vi "Producer Consumer Template.vi"   [LabVIEW 2020, in "Publisher Subscriber.lvlib"]
uses:
  Publisher Subscriber.lvlib
  Controls/node refnum.ctl
  Controls/data cluster.ctl
  37c060d3-9079-425a-9318-d9bb7186e347.vi
  ae88ff53-e2b6-4b5a-85aa-5b466751ef77.vi
types:
  T1 = typedef "Publisher Subscriber.lvlib/node refnum.ctl" = refnum<k1>
  T2 = cluster{"Node Ref":T1, "E Ref":refnum<event-registration>, "Message":string, "Tout":i32}
  T3 = cluster{"Node Ref":T1, "Message":string, "Tout":i32}
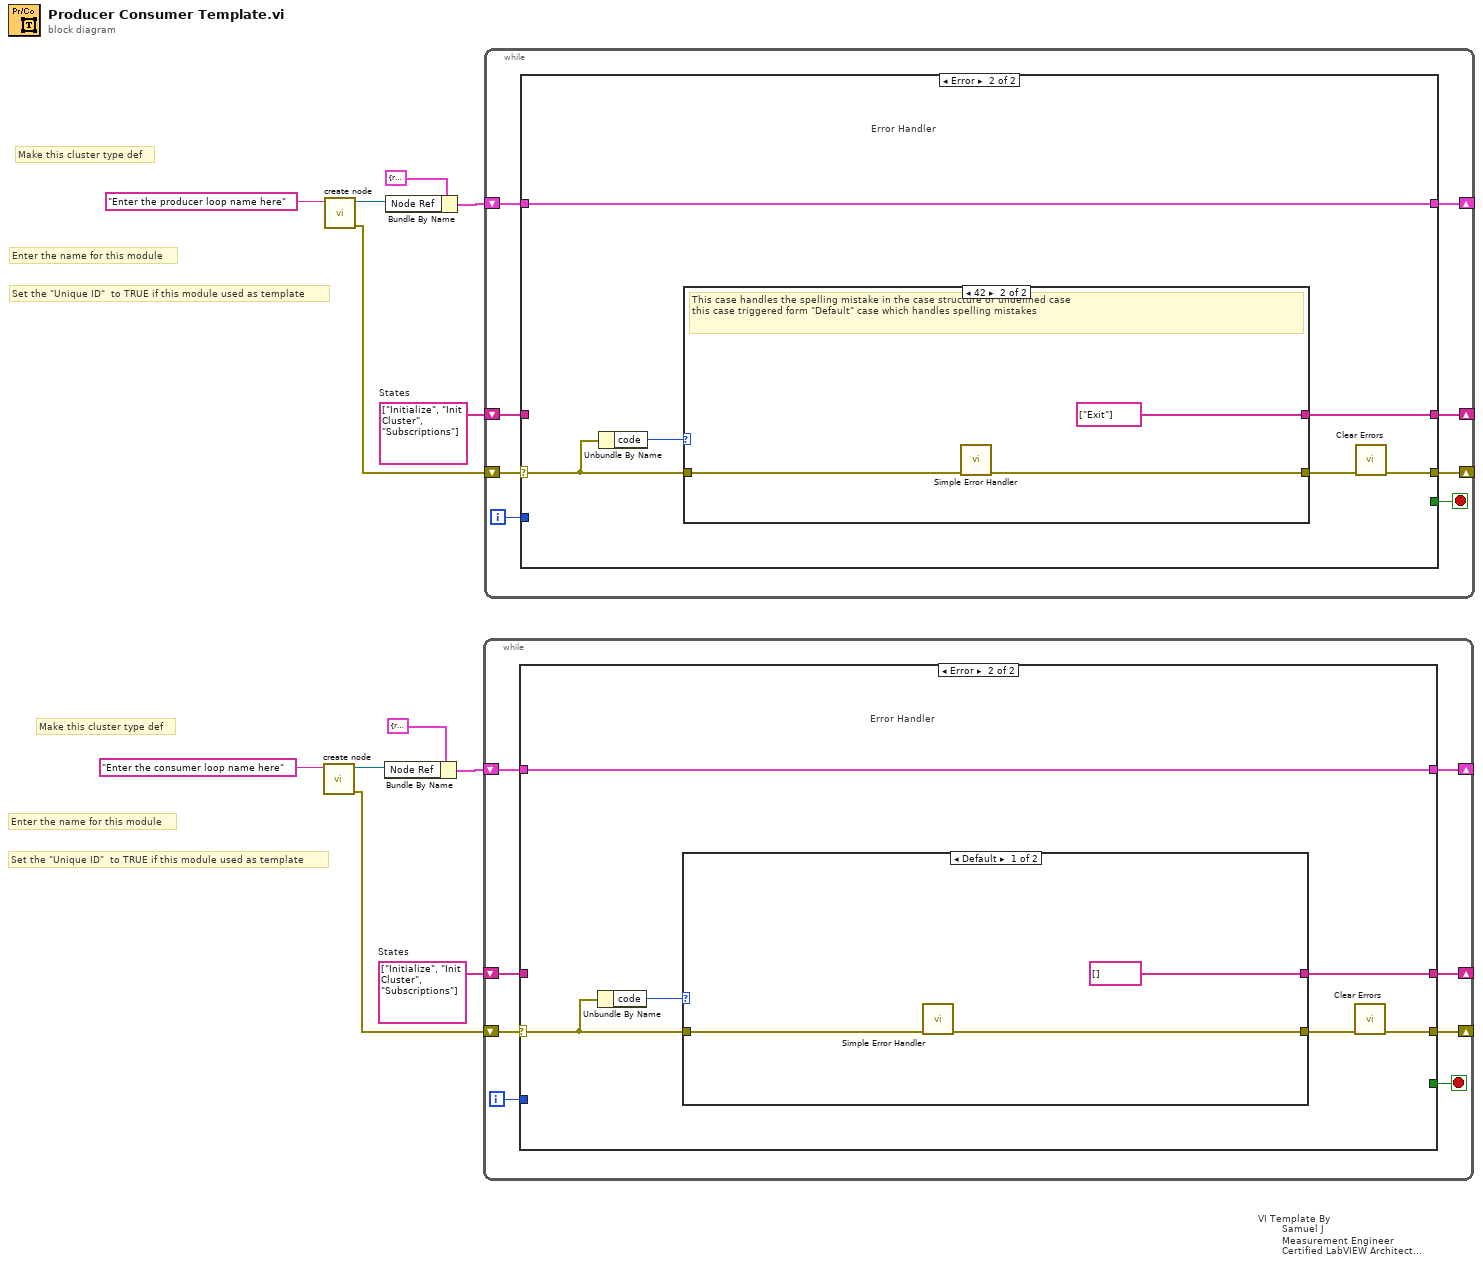
[diagram p0: block diagram]
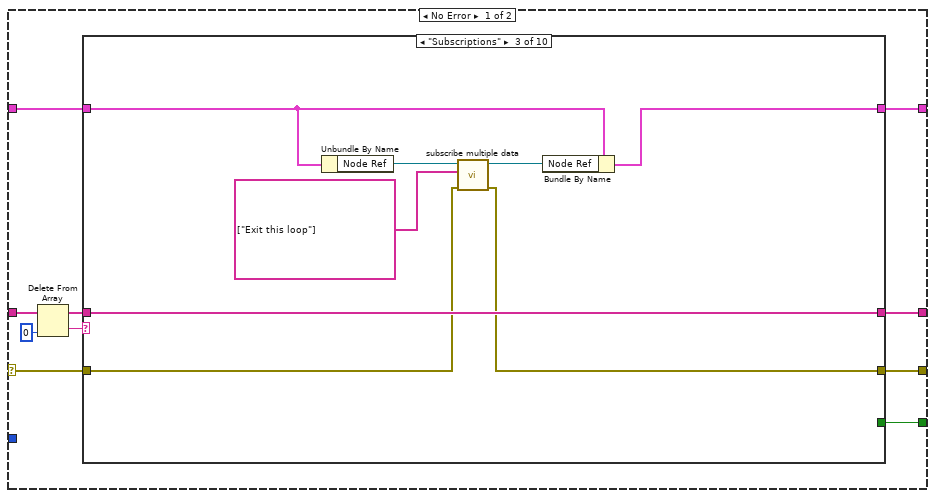
[diagram p2: hidden frame]
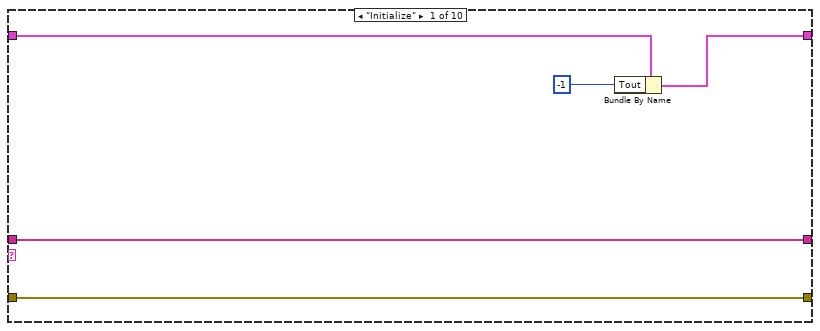
[diagram p3: hidden frame]
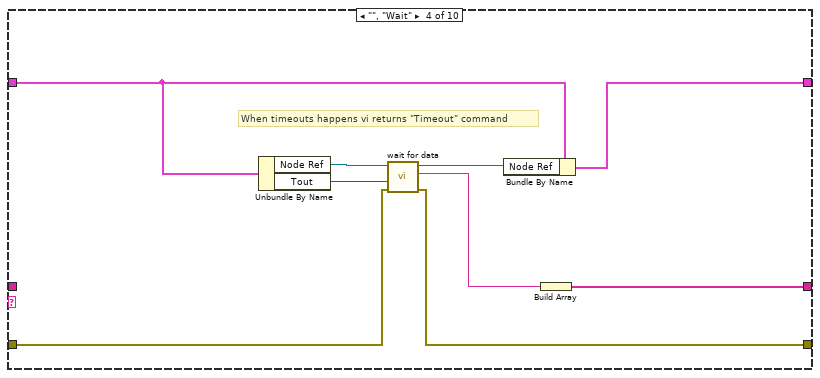
[diagram p5: hidden frame]
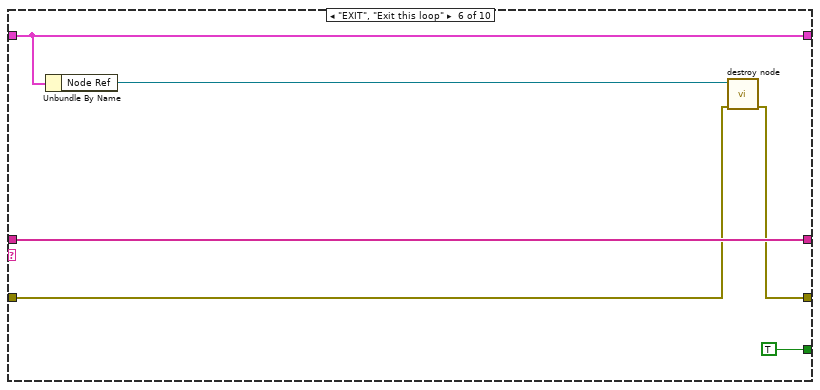
[diagram p7: hidden frame]
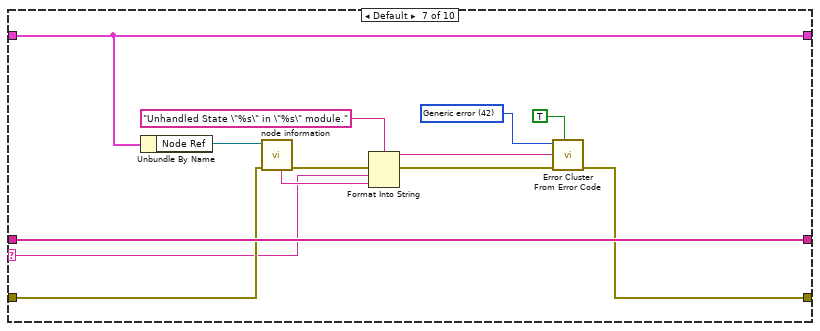
[diagram p8: hidden frame]
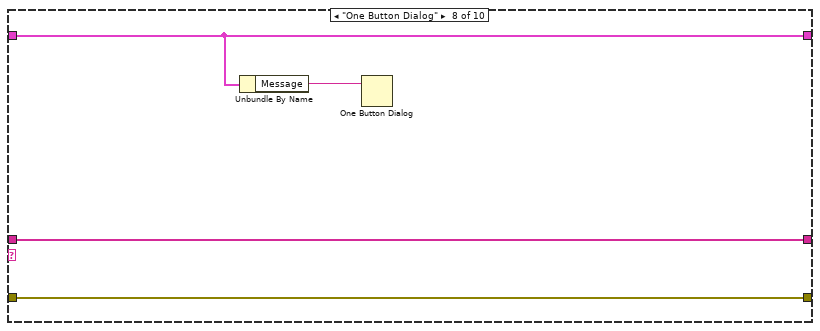
[diagram p9: hidden frame]
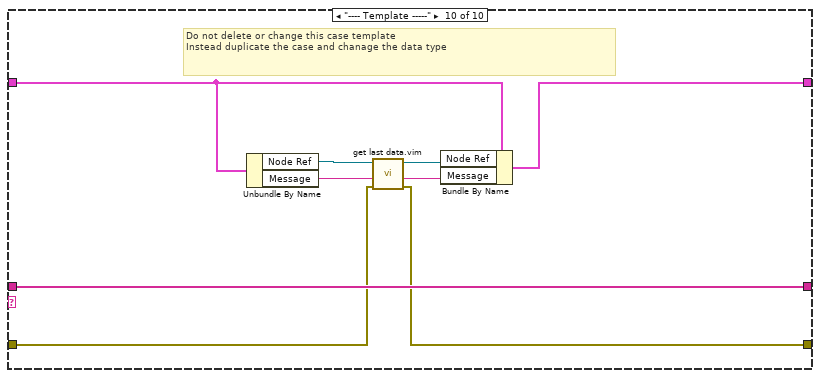
[diagram p11: hidden frame]
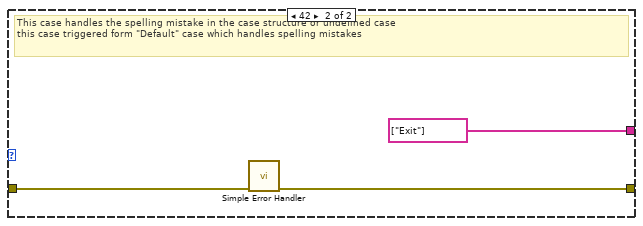
[diagram p12: hidden frame]
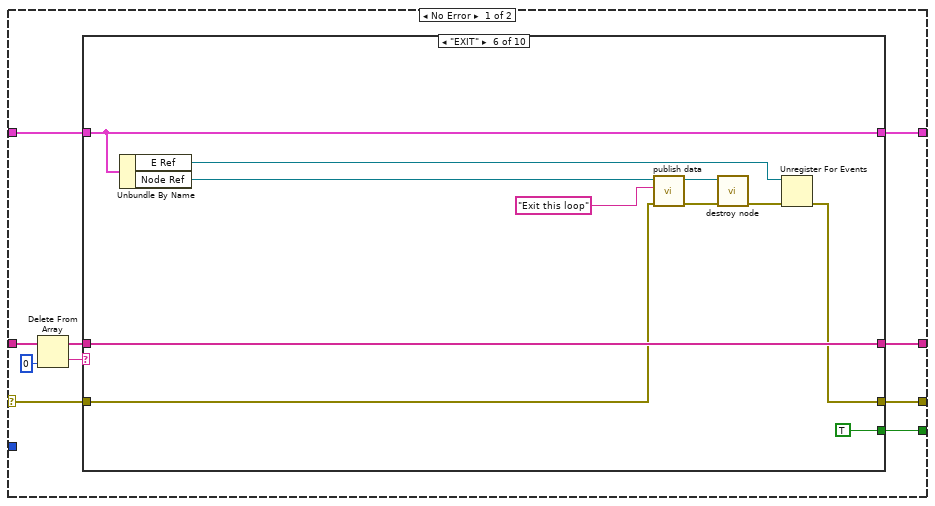
[diagram p13: hidden frame]
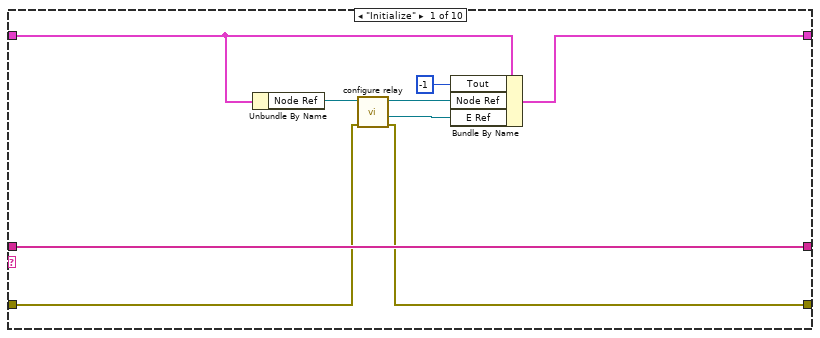
[diagram p14: hidden frame]
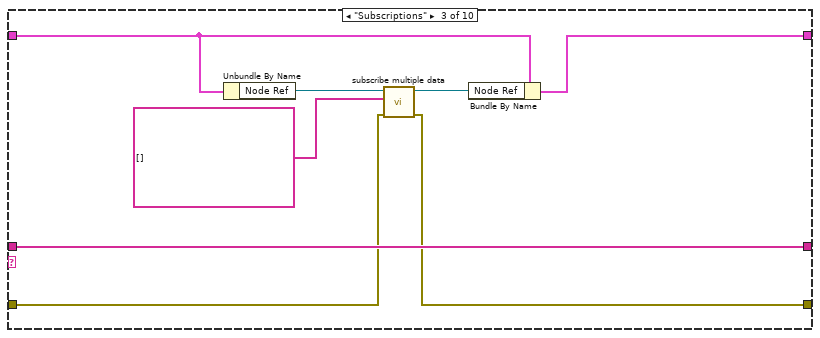
[diagram p16: hidden frame]
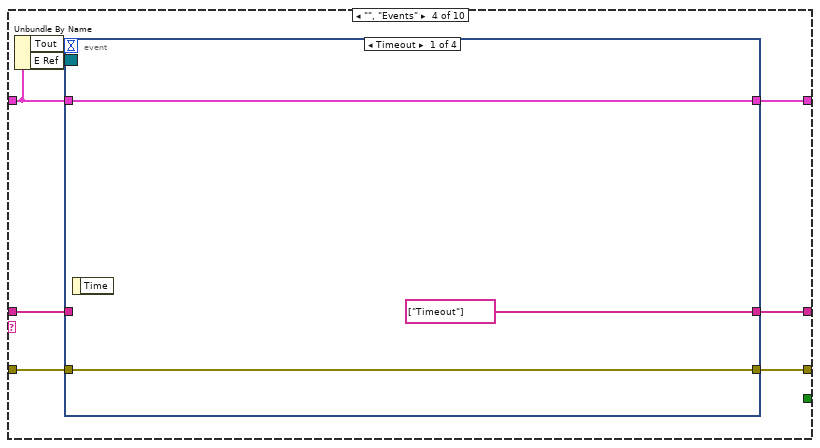
[diagram p17: hidden frame]
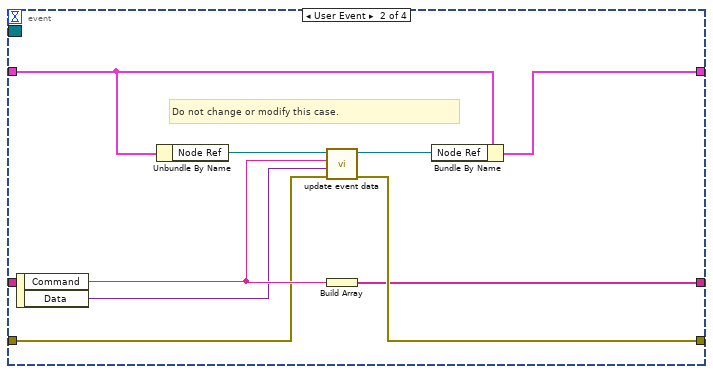
[diagram p18: hidden frame]
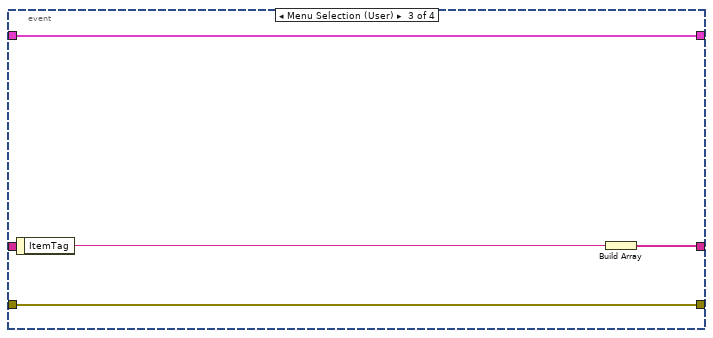
[diagram p19: hidden frame]
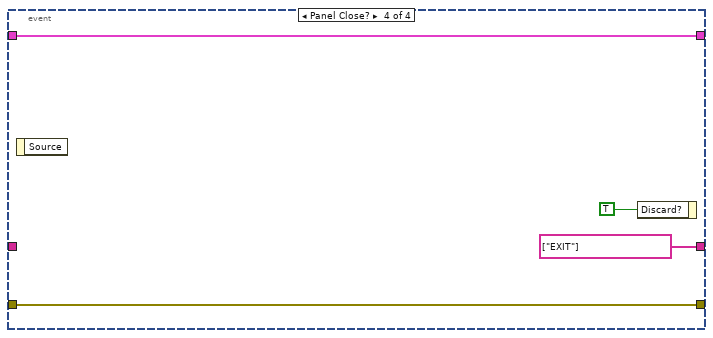
[diagram p20: hidden frame]
diagram:
  w6 = string[] ["Initialize", "Init Cluster", "Subscriptions"]  # States
  w12 = string[] ["Initialize", "Init Cluster", "Subscriptions"]  # States
  # "Set the \"Unique ID\"  to TRUE if this module used as template"
  # "Enter the name for this module"
  # "Make this cluster type def"
  # "Set the \"Unique ID\"  to TRUE if this module used as template"
  # "Enter the name for this module"
  # "Make this cluster type def"
  n1 = call "create node.vi"("node name"="Enter the consumer loop name here" ("Subscriber name")) -> ("error out"=w7:errorcluster, "node ref out"=w9:T1)  [unwired: 9 in]
  n2 = call "create node.vi"("node name"="Enter the producer loop name here" ("Subscriber name")) -> ("error out"=w1:errorcluster, "node ref out"=w3:T1)  [unwired: 9 in]
  n3 = Bundle By Name(cluster=T3 {"Node Ref"=refnum, "Message"="", "Tout"=-1} ("Cluster"), "Node Ref"=w9) -> (w10:T3)
  n4 = Bundle By Name(cluster=T2 {"Node Ref"=refnum, "E Ref"=refnum, "Message"="", "Tout"=-1} ("Cluster"), "Node Ref"=w3) -> (w4:T2)
  n5 = while "VI Template By\n        Samuel J\n        Measurement Engineer\n        Certified LabVIEW Architect\n        Vestas Technology R&D Chennai" {
    shift-right: [w16] -> _
    shift-left: w12 -> [w20]
    shift-right: [w17] -> _
    shift-left: w7 -> [w19]
    shift-right: [w15] -> _
    shift-left: w10 -> [w18]
    i -> [w13]
    stop <- w14 stop-if-true
    n6 = case shown="Error" w19 {
      selector: w19 -> [w25 w97]
      tunnel: w20 -> [w29 _]
      tunnel: w18 -> [w26 w99]
      tunnel: [w24 w95] -> w17
      tunnel: [w23 w94] -> w16
      tunnel: [w22 w99] -> w15
      tunnel: [w21 _] -> w14
      tunnel: w13 -> [_ _]
      frame No Error {
        n7 = Delete From Array(array=w29, index=0) -> (deleted portion=w28:string, array with subset deleted=w27:string[])  [unwired: 1 in]
        n8 = case shown="\"Subscriptions\"" w28 {
          selector: w28 -> [_ _ _ _ _ _ w66 _ _ _]
          tunnel: w27 -> [w35 w37 w46 _ w57 w64 w77 w79 w83 w93]
          tunnel: w26 -> [w33 w36 w43 w54 w56 w61 w68 w78 w82 w90]
          tunnel: w25 -> [w31 w38 w40 w52 w58 w59 w67 w80 w84 w87]
          tunnel: [w31 w38 w41 w50 w58 w60 w65 w80 w84 w88] -> w24
          tunnel: [w35 w37 w46 w48 w57 w64 w77 w79 w83 w93] -> w23
          tunnel: [w34 w36 w44 w47 w56 w61 w68 w78 w82 w91] -> w22
          tunnel: [_ _ _ _ _ TRUE ("Exit") _ _ _ _] -> w21
          frame "Initialize" {
            n9 = Bundle By Name(cluster=w33, "Tout"=-1) -> (w34:T3)
          }
          frame "Init Cluster" {
          }
          frame "Subscriptions" {
            n10 = Unbundle By Name(w43) -> ("Node Ref"=w45:T1)
            n11 = call "subscribe multiple data.vi"("error in"=w40, "subriscription list[]"=string[] ["Exit this loop"], "refnum in"=w45) -> ("error out"=w41:errorcluster, "refnum out"=w42:T1)  [unwired: 7 in]
            n12 = Bundle By Name(cluster=w43, "Node Ref"=w42) -> (w44:T3)
          }
          frame "", "Wait" {
            # "When timeouts happens vi returns \"Timeout\" command"
            n13 = Unbundle By Name(w54) -> ("Node Ref"=w55:T1, "Tout"=w53:i32)
            n14 = call "wait for data.vi"("error in"=w52, "timeout in ms (-1)"=w53, "refnum in"=w55) -> ("error out"=w50:errorcluster, "command"=w49:string, "refnum out"=w51:T1)  [unwired: 5 in, 1 out]
            n15 = Bundle By Name(cluster=w54, "Node Ref"=w51) -> (w47:T3)
            n16 = Build Array(w49) -> (w48:string[])
          }
          frame "Timeout" {
            # "Do not delete this case. Add your timeout code here else leave as it is."
          }
          frame "EXIT", "Exit this loop" {
            n17 = Unbundle By Name(w61) -> ("Node Ref"=w62:T1)
            n18 = call "destroy node.vi"("error in"=w59, "refnum in"=w62) -> ("error out"=w60:errorcluster)  [unwired: 8 in, 1 out]
          }
          frame Default {
            w73 = 42 items=["No error", "Argument error", "Memory is full", "Out of zone", "End of file", "File already open", "Generic file I/O error", "File not found", "File permission error", "Disk is full", "Duplicate path", "Too many files open", "System feature not enabled", "Resource file not found", "Cannot add resource", "Resource not found", "Image not found", "Image memory error", "Pen does not exist", "Config type invalid", "Config token not found", "Config parse error", "Config memory error", "Bad external code format", "Bad external code offset", "External code not present", "Null window", "Destroy window error", "Null menu", "Print aborted", "Bad print record", "Print driver error", "Windows error during printing", "Memory error during printing", "Print dialog error", "Generic print error", "Invalid device refnum", "Device not found", "Device parameter error", "Device unit error", "Cannot open device", "Device call aborted", "Generic error", "Cancelled by user", "Object ID too low", "Object ID too high", "Object not in heap", "Unknown heap", "Unknown object (invalid DefProc)", "Unknown object (DefProc not in table)", "Message out of range", "Invalid (null) method", "Unknown message", "Manager call not supported", "Bad address", "Network operation in progress", "Network operation timed out", "Connection is busy", "Network attribute not supported", "Network error", "Address in use", "System out of memory", "Connection aborted", "Connection refused", "Not connected", "Already connected", "Connection closed", "Initialization error (interapplication manager)", "Bad occurrence", "Wait on unbound occurrence handler", "Occurrence queue overflow", "Datalog type conflict", "Unused", "Unrecognized type (interapplication manager)", "Memory corrupt", "Failed to make temporary DLL", "Old CIN version", "Drag socket not found", "Failed to load drop-object", "Failed to register OLE object", "Failed to release OLE object", "Format specifier type mismatch", "Unknown format specifier", "Too few format specifiers", "Too many format specifiers", "Scan failed", "Newer CIN version", "Error converting to variant", "Runtime menu error", "Password tampered", "Variant attribute not found", "Incompatible variant data type", "Event data is not available", "Event Store is not present", "Occurrence is not found", "Event Queue is not created", "Event info is not available", "Refnum passed is NULL", "Error retrieving Class GUID", "Error retrieving CoClass GUID", "Error retrieving TypeLib GUID.", "Bad built application magic bytes.", "Specific driver is different from the specific driver associated with the Logical Name.", "There is no session opened to the class driver.", "Max Error", "MAX - Error with config objects", "MAX - Error loading configuration", "MAX - Group not supported"]
            n19 = Unbundle By Name(w68) -> ("Node Ref"=w71:T1)
            n20 = call "node information.vi"("error in"=w67, "refnum in"=w71) -> ("error out"=w69:errorcluster, "this node name"=w70:string)  [unwired: 4 in, 4 out]
            n21 = Format Into String(format string="Unhandled State \"%s\" in \"%s\" module." ("message"), error in=w69, w66, w70) -> (resulting string=w74:string, error out=w75:errorcluster)  [unwired: 1 in]
            n22 = call <vilib>:"Error Cluster From Error Code.vi"("show call chain? (False)"=TRUE, "error in (no error)"=w75, "error message (\"\")"=w74, "error code (0)"=w73) -> ("error out"=w65:errorcluster)  [unwired: 5 out]
          }
          frame "One Button Dialog" {
            n23 = Unbundle By Name(w78) -> ("Message"=w81:string)
            n24 = One Button Dialog(message=w81) -> ()  [unwired: 2 out]
          }
          frame "======== DATA =========" {
          }
          frame "---- Template -----" {
            # "Do not delete or change this case template \nInstead duplicate the case and chanage the data type"
            n25 = Unbundle By Name(w90) -> ("Node Ref"=w92:T1, "Message"=w86:string)
            n26 = call "get last data.vim"("error in"=w87, "data type"=w86, "refnum in"=w92) -> ("error out"=w88:errorcluster, "data out"=w85:string, "refnum out"=w89:T1)  [unwired: 5 in, 1 out]
            n27 = Bundle By Name(cluster=w90, "Node Ref"=w89, "Message"=w85) -> (w91:T3)
          }
        }
      }
      frame Error {
        # "Error Handler"
        n28 = Unbundle By Name(w97) -> ("code"=w98:i32)
        n29 = case shown="Default" w98 {
          tunnel: w97 -> [w102 w105]
          tunnel: [w101 w104] -> w96
          tunnel: [string[] [] ("States") string[] ["Exit"] ("States")] -> w94
          frame Default {
            n30 = call <vilib>:"Simple Error Handler.vi"("error in (no error)"=w102) -> ("error out"=w101:errorcluster)  [unwired: 1 in, 7 out]
          }
          frame 42 {
            # "This case handles the spelling mistake in the case structure or undefined case\nthis case triggered form \"Default\" case which handles spelling mistakes"
            n31 = call <vilib>:"Simple Error Handler.vi"("error in (no error)"=w105) -> ("error out"=w104:errorcluster)  [unwired: 1 in, 7 out]
          }
        }
        n32 = call <vilib>:"Clear Errors.vi"("error in (no error)"=w96) -> ("error out"=w95:errorcluster)  [unwired: 1 in, 5 out]
      }
    }
  }
  n33 = while "VI Template By\n        Samuel J\n        Measurement Engineer\n        Certified LabVIEW Architect\n        Vestas Technology R&D Chennai" {
    shift-right: [w109] -> _
    shift-left: w6 -> [w113]
    shift-right: [w110] -> _
    shift-left: w1 -> [w112]
    shift-right: [w108] -> _
    shift-left: w4 -> [w111]
    i -> [w106]
    stop <- w107 stop-if-true
    n34 = case shown="Error" w112 {
      selector: w112 -> [w118 w218]
      tunnel: w113 -> [w122 _]
      tunnel: w111 -> [w119 w220]
      tunnel: [w117 w216] -> w110
      tunnel: [w116 w215] -> w109
      tunnel: [w115 w220] -> w108
      tunnel: [w114 _] -> w107
      tunnel: w106 -> [_ _]
      frame No Error {
        n35 = Delete From Array(array=w122, index=0) -> (deleted portion=w121:string, array with subset deleted=w120:string[])  [unwired: 1 in]
        n36 = case shown="\"EXIT\"" w121 {
          selector: w121 -> [_ _ _ _ _ _ w192 _ _ _]
          tunnel: w120 -> [w132 w134 w143 w147 w173 w185 w198 w200 w204 w214]
          tunnel: w119 -> [w129 w133 w140 w146 w172 w183 w190 w199 w203 w211]
          tunnel: w118 -> [w126 w135 w137 w151 w174 w178 w186 w201 w205 w208]
          tunnel: [w127 w135 w138 w149 w174 w175 w191 w201 w205 w209] -> w117
          tunnel: [w132 w134 w143 w148 w173 w185 w198 w200 w204 w214] -> w116
          tunnel: [w130 w133 w141 w150 w172 w183 w190 w199 w203 w212] -> w115
          tunnel: [_ _ _ _ _ TRUE ("Exit") _ _ _ _] -> w114
          frame "Initialize" {
            n37 = Unbundle By Name(w129) -> ("Node Ref"=w131:T1)
            n38 = call "configure relay.vi"("error in"=w126, "Node Ref in"=w131) -> ("error out"=w127:errorcluster, "Event Reg Ref"=w124:refnum<event-registration>, "Node Ref out"=w128:T1)  [unwired: 7 in]
            n39 = Bundle By Name(cluster=w129, "Tout"=-1, "Node Ref"=w128, "E Ref"=w124) -> (w130:T2)
          }
          frame "Init Cluster" {
          }
          frame "Subscriptions" {
            n40 = Unbundle By Name(w140) -> ("Node Ref"=w142:T1)
            n41 = call "subscribe multiple data.vi"("error in"=w137, "subriscription list[]"=string[] [], "refnum in"=w142) -> ("error out"=w138:errorcluster, "refnum out"=w139:T1)  [unwired: 7 in]
            n42 = Bundle By Name(cluster=w140, "Node Ref"=w139) -> (w141:T2)
          }
          frame "", "Events" {
            n43 = Unbundle By Name(w146) -> ("Tout"=w144:i32, "E Ref"=w145:refnum<event-registration>)
            n44 = event shown="[0] Timeout" {
              selector: w145 -> [_ _ _ _]
              dyn-events: _ -> [_ _ _ _]
              timeout: w144 -> [_ _ _ _]
              tunnel: w146 -> [w154 w156 w167 w170]
              tunnel: w151 -> [w153 w159 w164 w169]
              tunnel: [w154 w155 w167 w170] -> w150
              tunnel: [w153 w158 w164 w169] -> w149
              tunnel: [string[] ["Timeout"] ("States") w157 w165 string[] ["EXIT"] ("States")] -> w148
              tunnel: w147 -> [_ _ _ _]
              event Timeout {
                n45 = event-data() -> ()  [unwired: 2 out]
              }
              event User Event {
                # "Do not change or modify this case."
                n46 = event-data() -> ("Command"=w161:string, "Data"=w160:variant)  [unwired: 1 out]
                n47 = Unbundle By Name(w156) -> ("Node Ref"=w163:T1)
                n48 = call "update event data.vi"("error in"=w159, "data type"=w160, "Command"=w161, "refnum in"=w163) -> ("error out"=w158:errorcluster, "refnum in"=w162:T1)  [unwired: 6 in]
                n49 = Build Array(w161) -> (w157:string[])
                n50 = Bundle By Name(cluster=w156, "Node Ref"=w162) -> (w155:T2)
              }
              event Menu Selection (User) {
                n51 = event-data() -> ("ItemTag"=w166:string)  [unwired: 1 out]
                n52 = Build Array(w166) -> (w165:string[])
              }
              event Panel Close? {
                n53 = event-data() -> ()  [unwired: 2 out]
                n54 = event-data("Discard?"=TRUE) -> ()  [unwired: 1 in, 1 out]
              }
            }
          }
          frame "Timeout" {
            # "Do not delete this case. Add your timeout code here else leave as it is."
          }
          frame "EXIT" {
            n55 = Unbundle By Name(w183) -> ("E Ref"=w177:refnum<event-registration>, "Node Ref"=w182:T1)
            n56 = call "publish data.vi"("error in"=w178, "command"="Exit this loop", "refnum in"=w182) -> ("error out"=w180:errorcluster, "refnum out"=w181:T1)  [unwired: 7 in]
            n57 = call "destroy node.vi"("error in"=w180, "refnum in"=w181) -> ("error out"=w176:errorcluster)  [unwired: 8 in, 1 out]
            n58 = Unregister For Events(event registration refnum=w177, error in=w176) -> (error out=w175:errorcluster)
          }
          frame Default {
            w194 = 42 items=["No error", "Argument error", "Memory is full", "Out of zone", "End of file", "File already open", "Generic file I/O error", "File not found", "File permission error", "Disk is full", "Duplicate path", "Too many files open", "System feature not enabled", "Resource file not found", "Cannot add resource", "Resource not found", "Image not found", "Image memory error", "Pen does not exist", "Config type invalid", "Config token not found", "Config parse error", "Config memory error", "Bad external code format", "Bad external code offset", "External code not present", "Null window", "Destroy window error", "Null menu", "Print aborted", "Bad print record", "Print driver error", "Windows error during printing", "Memory error during printing", "Print dialog error", "Generic print error", "Invalid device refnum", "Device not found", "Device parameter error", "Device unit error", "Cannot open device", "Device call aborted", "Generic error", "Cancelled by user", "Object ID too low", "Object ID too high", "Object not in heap", "Unknown heap", "Unknown object (invalid DefProc)", "Unknown object (DefProc not in table)", "Message out of range", "Invalid (null) method", "Unknown message", "Manager call not supported", "Bad address", "Network operation in progress", "Network operation timed out", "Connection is busy", "Network attribute not supported", "Network error", "Address in use", "System out of memory", "Connection aborted", "Connection refused", "Not connected", "Already connected", "Connection closed", "Initialization error (interapplication manager)", "Bad occurrence", "Wait on unbound occurrence handler", "Occurrence queue overflow", "Datalog type conflict", "Unused", "Unrecognized type (interapplication manager)", "Memory corrupt", "Failed to make temporary DLL", "Old CIN version", "Drag socket not found", "Failed to load drop-object", "Failed to register OLE object", "Failed to release OLE object", "Format specifier type mismatch", "Unknown format specifier", "Too few format specifiers", "Too many format specifiers", "Scan failed", "Newer CIN version", "Error converting to variant", "Runtime menu error", "Password tampered", "Variant attribute not found", "Incompatible variant data type", "Event data is not available", "Event Store is not present", "Occurrence is not found", "Event Queue is not created", "Event info is not available", "Refnum passed is NULL", "Error retrieving Class GUID", "Error retrieving CoClass GUID", "Error retrieving TypeLib GUID.", "Bad built application magic bytes.", "Specific driver is different from the specific driver associated with the Logical Name.", "There is no session opened to the class driver.", "Max Error", "MAX - Error with config objects", "MAX - Error loading configuration", "MAX - Group not supported"]
            n59 = Unbundle By Name(w190) -> ("Node Ref"=w189:T1)
            n60 = call "node information.vi"("error in"=w186, "refnum in"=w189) -> ("error out"=w187:errorcluster, "this node name"=w188:string)  [unwired: 4 in, 4 out]
            n61 = Format Into String(format string="Unhandled State \"%s\" in \"%s\" module." ("message"), error in=w187, w192, w188) -> (resulting string=w195:string, error out=w196:errorcluster)  [unwired: 1 in]
            n62 = call <vilib>:"Error Cluster From Error Code.vi"("show call chain? (False)"=TRUE, "error in (no error)"=w196, "error message (\"\")"=w195, "error code (0)"=w194) -> ("error out"=w191:errorcluster)  [unwired: 5 out]
          }
          frame "One Button Dialog" {
            n63 = Unbundle By Name(w199) -> ("Message"=w202:string)
            n64 = One Button Dialog(message=w202) -> ()  [unwired: 2 out]
          }
          frame "======== DATA =========" {
          }
          frame "---- Template -----" {
            # "Do not delete or change this case template \nInstead duplicate the case and chanage the data type"
            n65 = Unbundle By Name(w211) -> ("Node Ref"=w213:T1, "Message"=w207:string)
            n66 = call "get last data.vim"("error in"=w208, "data type"=w207, "refnum in"=w213) -> ("error out"=w209:errorcluster, "data out"=w206:string, "refnum out"=w210:T1)  [unwired: 5 in, 1 out]
            n67 = Bundle By Name(cluster=w211, "Node Ref"=w210, "Message"=w206) -> (w212:T2)
          }
        }
      }
      frame Error {
        # "Error Handler"
        n68 = Unbundle By Name(w218) -> ("code"=w219:i32)
        n69 = case shown="42" w219 {
          tunnel: w218 -> [w223 w224]
          tunnel: [w222 w225] -> w217
          tunnel: [string[] [] ("States") string[] ["Exit"] ("States")] -> w215
          frame Default {
            n70 = call <vilib>:"Simple Error Handler.vi"("error in (no error)"=w223) -> ("error out"=w222:errorcluster)  [unwired: 1 in, 7 out]
          }
          frame 42 {
            # "This case handles the spelling mistake in the case structure or undefined case\nthis case triggered form \"Default\" case which handles spelling mistakes"
            n71 = call <vilib>:"Simple Error Handler.vi"("error in (no error)"=w224) -> ("error out"=w225:errorcluster)  [unwired: 1 in, 7 out]
          }
        }
        n72 = call <vilib>:"Clear Errors.vi"("error in (no error)"=w217) -> ("error out"=w216:errorcluster)  [unwired: 1 in, 5 out]
      }
    }
  }
